vi "Coverage Analyzer View.vi"(8 "error in (no error)":errorcluster, 11 "Coverage Analyzer Result View.lvclass":refnum<class "Coverage Analyzer Result View.lvclass">) -> (0 "error out":errorcluster)   [LabVIEW 2020, in "Coverage Analyzer.lvlib" / "Coverage Analyzer Result View.lvclass"]
uses:
  Coverage Analyzer Result View.lvclass
  Coverage Analyzer Result View.lvclass/Coverage Analyzer Result View.ctl
panel:
  in  "Method Test Times":i32(listbox)
  out "Debug disabled VIs":string
  out "Coverage for Executed VIs":string
  out "Fraction of VIs Executed":string
  in  "Hide VIs not executed?":bool=TRUE
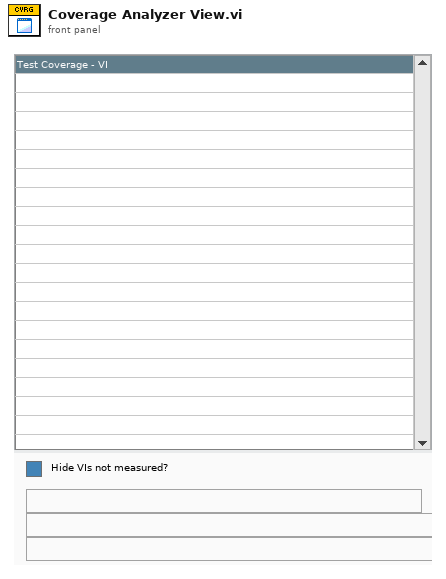
[diagram p1: front panel]
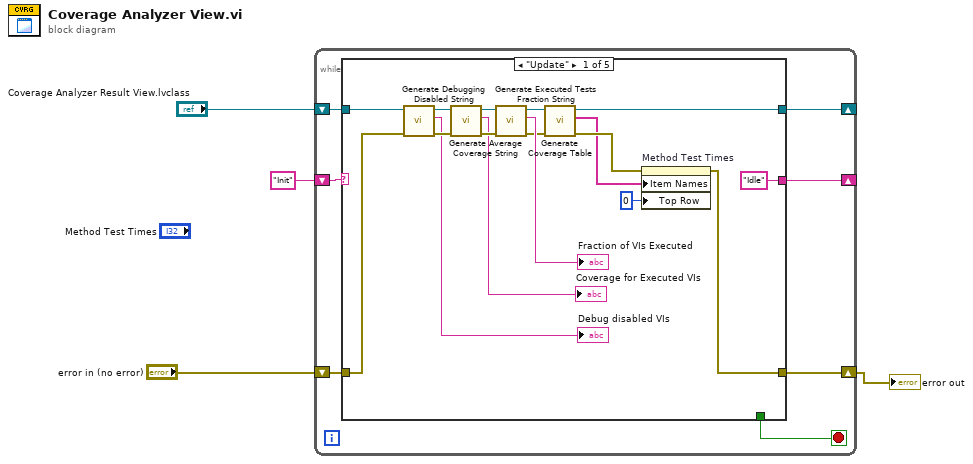
[diagram p0: block diagram]
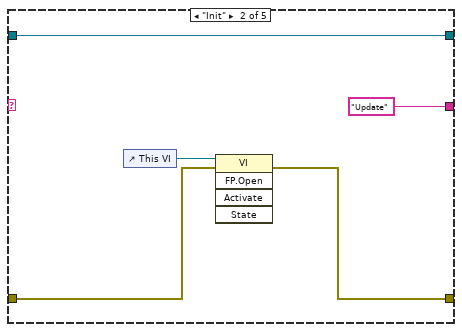
[diagram p2: hidden frame]
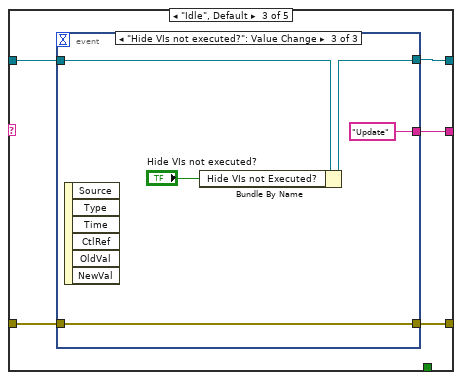
[diagram p3: hidden frame]
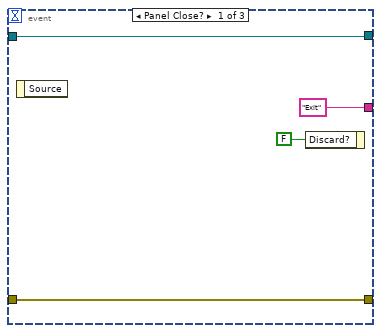
[diagram p4: hidden frame]
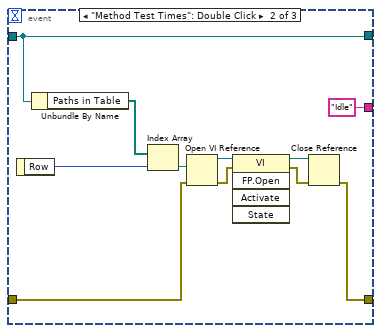
[diagram p5: hidden frame]
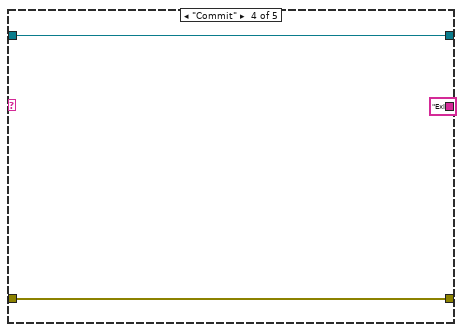
[diagram p6: hidden frame]
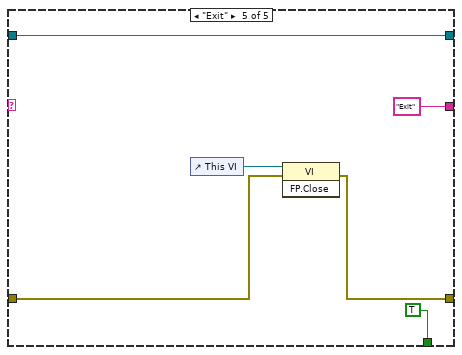
[diagram p7: hidden frame]
diagram:
  n1 = while {
    shift-right: [w8] -> _
    shift-left: "Coverage Analyzer Result View.lvclass" -> [w9]
    shift-right: [w5] -> w2
    shift-left: "error in (no error)" -> [w10]
    shift-right: [w7] -> _
    shift-left: "Init" -> [w11]
    stop <- w6 stop-if-true
    n2 = case shown="\"Update\"" w11 {
      tunnel: [w27 w31 w38 w61 w63] -> w5
      tunnel: w10 -> [w21 w30 w37 w61 w62]
      tunnel: w9 -> [w14 w29 w36 w60 w67]
      tunnel: [w24 w29 w35 w60 w67] -> w8
      tunnel: ["Idle" "Update" w34 "Exit" "Exit"] -> w7
      tunnel: [_ _ _ _ TRUE] -> w6
      frame "Update" {
        n3 = call "Generate Debugging Disabled String.vi"("error in (no error)"=w21, "Coverage Analyzer Result View in"=w14) -> ("error out"=w15:errorcluster, "Disabled Debuggin"=→"Debug disabled VIs":string, "Coverage Analyzer Result View out"=w13:refnum<class "Coverage Analyzer Result View.lvclass">)  [unwired: 7 in]
        n4 = call "Generate Average Coverage String.vi"("error in (no error)"=w15, "Coverage Analyzer Result View in"=w13) -> ("error out"=w19:errorcluster, "Fraction of VIs Executed"=→"Coverage for Executed VIs":string, "Coverage Analyzer Result View out"=w18:refnum<class "Coverage Analyzer Result View.lvclass">)  [unwired: 7 in]
        n5 = call "Generate Executed Tests Fraction String.vi"("error in (no error)"=w19, "Coverage Analyzer Result View in"=w18) -> ("error out"=w20:errorcluster, "Fraction of VIs Executed"=→"Fraction of VIs Executed":string, "Coverage Analyzer Result View out"=w22:refnum<class "Coverage Analyzer Result View.lvclass">)  [unwired: 7 in]
        n6 = call "Generate Coverage Table.vi"("error in (no error)"=w20, "Coverage Analyzer Result View In"=w22) -> ("error out"=w26:errorcluster, "Item Names"=w25:string[], "Coverage Analyzer Result View Out"=w24:refnum<class "Coverage Analyzer Result View.lvclass">)  [unwired: 7 in]
        n7 = property on="Method Test Times" class="LstBox (strict)"(error in=w26, "Item Names"=w25, "Top Row"=0) -> (error out=w27:errorcluster)  [unwired: 1 in, 1 out]
      }
      frame "Init" {
        n8 = control-ref of="This VI"() -> (w32:refnum<vi>)
        n9 = invoke class="VI" method="FP.Open"(reference=w32, error in=w30) -> (error out=w31:errorcluster)  [unwired: 3 in, 4 out]
      }
      frame "Idle", Default {
        n10 = event shown="[2] \"Hide VIs not executed?\": Value Change" {
          selector: _ -> [_ _ _]
          dyn-events: _ -> [_ _ _]
          timeout: _ -> [_ _ _]
          tunnel: [w42 w44 w58] -> w38
          tunnel: w37 -> [w42 w43 w58]
          tunnel: w36 -> [w41 w52 w57]
          tunnel: [w41 w52 w55] -> w35
          tunnel: ["Exit" "Idle" "Update"] -> w34
          event Panel Close? {
            n11 = event-data() -> ()  [unwired: 1 in, 1 out]
            n12 = event-data("Discard?"=FALSE) -> ()  [unwired: 1 in, 1 out]
          }
          event "Method Test Times": Double Click {
            n13 = event-data() -> ("Row"=w50:i32)  [unwired: 1 in]
            n14 = Unbundle By Name(w52) -> ("Paths in Table"=w51:path[])
            n15 = Index Array(array=w51, index=w50) -> (element=w49:path)
            n16 = Open VI Reference(vi path=w49, error in (no error)=w43) -> (vi reference=w48:refnum<vi>, error out=w47:errorcluster)  [unwired: 4 in]
            n17 = invoke class="VI" method="FP.Open"(reference=w48, error in=w47) -> (reference out=w46:refnum<vi>, error out=w45:errorcluster)  [unwired: 3 in, 3 out]
            n18 = Close Reference(reference=w46, error in (no error)=w45) -> (error out=w44:errorcluster)
          }
          event "Hide VIs not executed?": Value Change {
            n19 = event-data() -> ()  [unwired: 1 in, 6 out]
            n20 = Bundle By Name(cluster=w57, "Hide VIs not Executed?"="Hide VIs not executed?") -> (w55:refnum<class "Coverage Analyzer Result View.lvclass">)
          }
        }
      }
      frame "Commit" {
      }
      frame "Exit" {
        n21 = control-ref of="This VI"() -> (w64:refnum<vi>)
        n22 = invoke class="VI" method="FP.Close"(reference=w64, error in=w62) -> (error out=w63:errorcluster)  [unwired: 1 in, 2 out]
      }
    }
  }
  "error out" <- w2
